vi "Skip Value.vi"(8 "How Many?":i32, 11 "string in":string) -> (3 "string out":string)   [LabVIEW 2018]
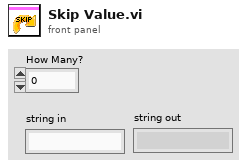
[diagram p1: front panel]
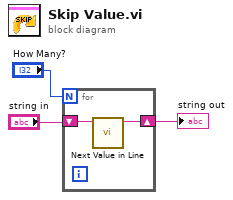
[diagram p0: block diagram]
diagram:
  n1 = for {
    N: "How Many?" -> [_]
    shift-right: [w4] -> w1
    shift-left: "string in" -> [w5]
    n2 = call "Next Value in Line.vi"("string in"=w5) -> ("rest of string"=w4:string)  [unwired: 9 in, 1 out]
  }
  "string out" <- w1
